vi "Read Config.vi"(8 "error in (no error)":errorcluster, 9 "Re-Init?":bool, 10 "ICM File In":path, 11 "Single Query in":refnum<class "Single Query.lvclass">) -> (0 "error out":errorcluster, 3 "Single Query out":refnum<class "Single Query.lvclass">)   [LabVIEW 2015, in "Single Query.lvclass"]
doc: "Single Query.lvclass:Read Config.vi\n\nThis VI reads the configuration data for the Single Query child class.\n\nInstrument Communication Module Version 1.0\nDecember, 2017 Original Code Consulting David Thomson\n www.originalcode.com"
uses:
  Single Query.lvclass
  Single Query.lvclass/Single Query.ctl
  Query/Query.lvclass
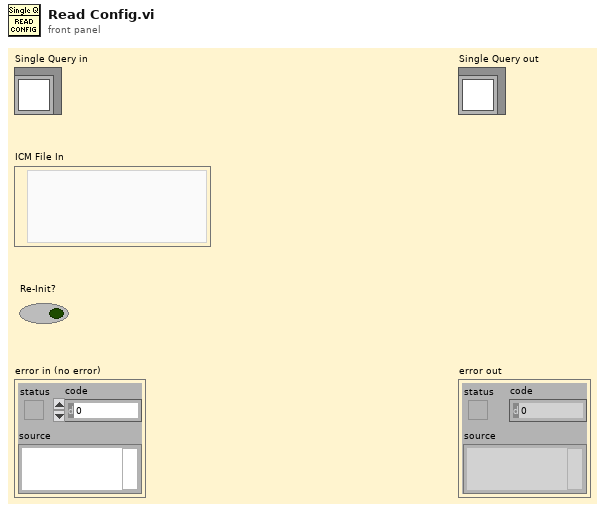
[diagram p1: front panel]
types:
  T1 = typedef "Single Query.lvclass/Single Query Config.ctl" = cluster{"Query String":string}
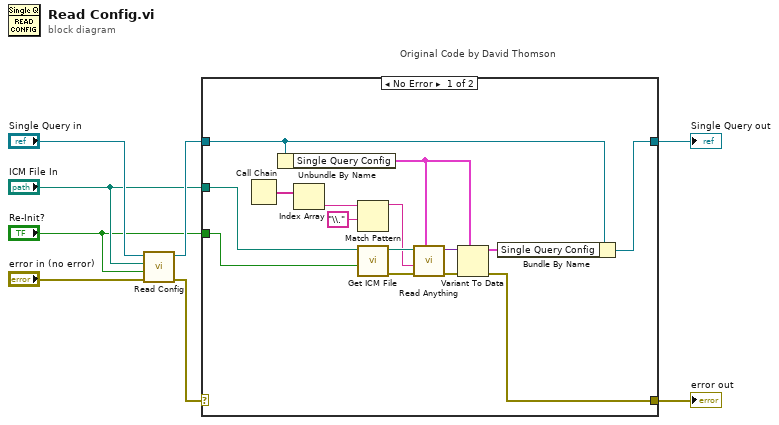
[diagram p0: block diagram]
diagram:
  n1 = call-parent "Read Config.vi"("error in (no error)"="error in (no error)", "Re-Init?"="Re-Init?", "ICM File In"="ICM File In", "Query in"="Single Query in") -> ("error out"=w6:errorcluster, "Query out"=w5:refnum<class "Single Query.lvclass">)  [unwired: 6 in]
  n2 = case "Original Code by David Thomson" shown="No Error" w6 {
    selector: w6 -> [_ w25]
    tunnel: [w15 w25] -> w1
    tunnel: [w12 w24] -> w2
    tunnel: w5 -> [w11 w24]
    tunnel: "ICM File In" -> [w10 _]
    tunnel: "Re-Init?" -> [w9 _]
    frame No Error {
      n3 = Call Chain() -> (call chain=w20:string[])
      n4 = Unbundle By Name(w11) -> ("Single Query Config"=w13:T1)
      n5 = Index Array(array=w20) -> (element=w21:string)  [unwired: 1 in]
      n6 = Match Pattern(string=w21, regular expression="\\.") -> (before substring=w18:string)  [unwired: 1 in, 3 out]
      n7 = call "Get ICM File.vi"("Re-Init?"=w9, "ICM File In"=w10) -> ("error out"=w22:errorcluster, "ICM File"=w23:path)  [unwired: 8 in]
      n8 = call "Read Anything.vi"("Type of Anything"=w13, "Error In"=w22, "Section Name (Name of \"Type of Anything\")"=w18, "Path (dialog)"=w23) -> ("Error Out"=w16:errorcluster, "Anything"=w17:variant)  [unwired: 5 in, 1 out]
      n9 = Variant To Data(error in=w16, type=w13, Variant=w17) -> (data=w14:T1, error out=w15:errorcluster)
      n10 = Bundle By Name(cluster=w11, "Single Query Config"=w14) -> (w12:refnum<class "Single Query.lvclass">)
    }
    frame Error {
    }
  }
  "error out" <- w1
  "Single Query out" <- w2
